vi "FourGaussiansNlin.vi"() -> ()   [LabVIEW 2015]
uses:
  <vilib>/gmath/NumericalOptimization/Nonlinear Curve Fit LM.vi
  <vilib>/gmath/NI_Gmath.lvlib
panel:
  out "array":dbl[][](array[numeric])
  out "error out":errorcluster
  in  "Parameter Guess":dbl[][](array[numeric])=[[1.0, 3224.0, 82.8], [1.0, 3280.0, 64.0], [1.0, 3480.0, 40.0], [1.0, 3518.0, 40.0]] caption="Amplitude     Position        Width" format="%.2f"
  out "Results":string[][](table)
  out "Fit":cluster{dbl, dbl, dbl[][]}(graph)
  # "Initial Guesses (add or remove rows as needed)"
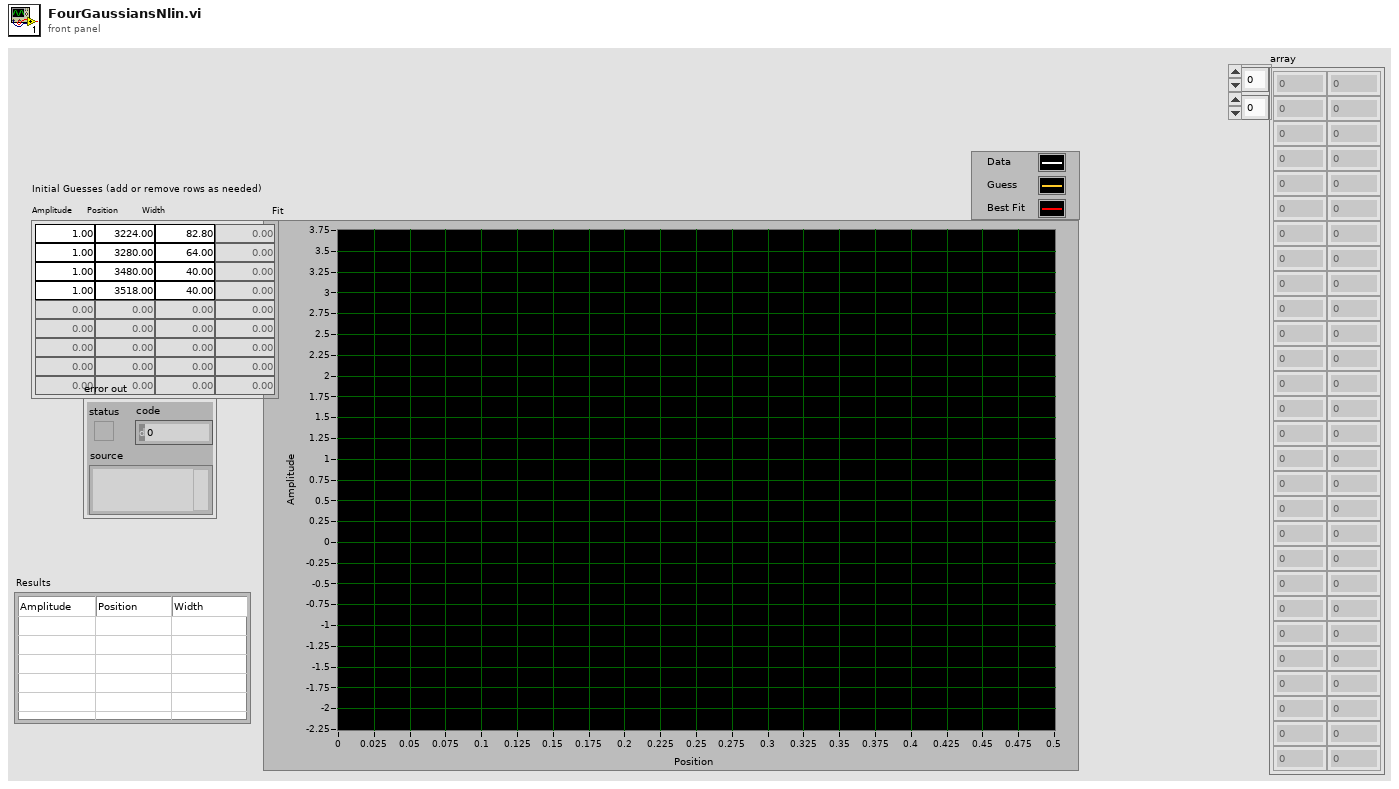
[diagram p1: front panel]
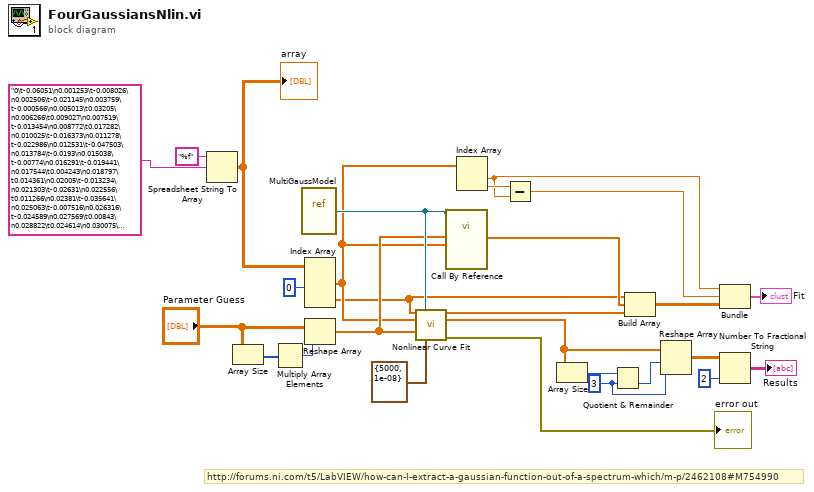
[diagram p0: block diagram]
diagram:
  w4 = 3 ("y")
  # "http://forums.ni.com/t5/LabVIEW/how-can-I-extract-a-gaussian-function-out-of-a-spectrum-which/m-p/2462108#M754990"
  n1 = Spreadsheet String To Array(format string="%f", spreadsheet string="0\t-0.06051\n0.001253\t-0.008026\n0.002506\t-0.021145\n0.003759\t-0.000566\n0.005013\t0.03205\n0.006266\t0.009027\n0.007519\t-0.013454\n0.008772\t0.017282\n0.010025\t-0.016373\n0.011278\t-0.022986\n0.012531\t-0.047503\n0.013784\t-0.0193\n0.015038\t-0.00774\n0.016291\t-0.019441\n0.017544\t0.004243\n0.018797\t0.014361\n0.02005\t-0.013234\n0.021303\t-0.02631\n0.022556\t0.011266\n0.02381\t-0.035641\n0.025063\t-0.007516\n0.026316\t-0.024589\n0.027569\t0.00843\n0.028822\t0.024614\n0.030075\t-0.045957\n0.031328\t-0.057716\n0.032581\t-0.043953\n0.033835\t-0.031529\n0.035088\t-0.081927\n0.036341\t-0.091408\n0.037594\t-0.098195\n0.038847\t-0.089564\n0.0401\t-0.038276\n0.041353\t-0.08202\n0.042607\t-0.091543\n0.04386\t-0.046757\n0.045113\t-0.09163\n0.046366\t-0.088749\n0.047619\t-0.064658\n0.048872\t-0.072261\n0.050125\t-0.12707\n0.051378\t-0.104708\n0.052632\t-0.103939\n0.053885\t-0.093157\n0.055138\t-0.132049\n0.056391\t-0.114817\n0.057644\t-0.121724\n0.058897\t-0.104782\n0.06015\t-0.142024\n0.061404\t-0.131957\n0.062657\t-0.176914\n0.06391\t-0.161334\n0.065163\t-0.14284\n0.066416\t-0.156644\n0.067669\t-0.201751\n0.068922\t-0.166965\n0.070175\t-0.188029\n0.071429\t-0.205835\n0.072682\t-0.272606\n0.073935\t-0.278951\n0.075188\t-0.27726\n0.076441\t-0.258719\n0.077694\t-0.230262\n0.078947\t-0.27264\n0.080201\t-0.295268\n0.081454\t-0.247801\n0.082707\t-0.284363\n0.08396\t-0.305459\n0.085213\t-0.322454\n0.086466\t-0.321781\n0.087719\t-0.361286\n0.088972\t-0.333156\n0.090226\t-0.348285\n0.091479\t-0.358595\n0.092732\t-0.39051\n0.093985\t-0.382925\n0.095238\t-0.491624\n0.096491\t-0.463605\n0.097744\t-0.462484\n0.098997\t-0.470019\n0.100251\t-0.469667\n0.101504\t-0.517955\n0.102757\t-0.59736\n0.10401\t-0.584936\n0.105263\t-0.577842\n0.106516\t-0.609382\n0.107769\t-0.595847\n0.109023\t-0.654391\n0.110276\t-0.651756\n0.111529\t-0.684239\n0.112782\t-0.675556\n0.114035\t-0.72925\n0.115288\t-0.712574\n0.116541\t-0.764648\n0.117794\t-0.74467\n0.119048\t-0.77396\n0.120301\t-0.829208\n0.121554\t-0.85807\n0.122807\t-0.902266\n0.12406\t-0.932697\n0.125313\t-0.898871\n0.126566\t-1.022656\n0.12782\t-0.929653\n0.129073\t-0.990668\n0.130326\t-1.016715\n0.131579\t-1.062086\n0.132832\t-1.088136\n0.134085\t-1.090147\n0.135338\t-1.178622\n0.136591\t-1.189203\n0.137845\t-1.158555\n0.139098\t-1.221042\n0.140351\t-1.225178\n0.141604\t-1.249981\n0.142857\t-1.296073\n0.14411\t-1.285886\n0.145363\t-1.310712\n0.146617\t-1.362254\n0.14787\t-1.366437\n0.149123\t-1.374629\n0.150376\t-1.408814\n0.151629\t-1.418909\n0.152882\t-1.461478\n0.154135\t-1.498747\n0.155388\t-1.530223\n0.156642\t-1.482521\n0.157895\t-1.561413\n0.159148\t-1.559136\n0.160401\t-1.651416\n0.161654\t-1.656585\n0.162907\t-1.606711\n0.16416\t-1.648703\n0.165414\t-1.657518\n0.166667\t-1.70666\n0.16792\t-1.780643\n0.169173\t-1.690411\n0.170426\t-1.798746\n0.171679\t-1.788852\n0.172932\t-1.84627\n0.174185\t-1.843477\n0.175439\t-1.833331\n0.176692\t-1.885198\n0.177945\t-1.887675\n0.179198\t-1.924923\n0.180451\t-1.874285\n0.181704\t-1.901879\n0.182957\t-1.907824\n0.184211\t-1.94076\n0.185464\t-1.952966\n0.186717\t-1.978324\n0.18797\t-1.97581\n0.189223\t-1.949066\n0.190476\t-2.007462\n0.191729\t-2.003745\n0.192982\t-2.002412\n0.194236\t-1.954237\n0.195489\t-1.968438\n0.196742\t-1.992692\n0.197995\t-1.998839\n0.199248\t-1.989507\n0.200501\t-1.948727\n0.201754\t-1.963294\n0.203008\t-1.96246\n0.204261\t-1.987921\n0.205514\t-1.928685\n0.206767\t-1.96992\n0.20802\t-1.970377\n0.209273\t-1.925754\n0.210526\t-1.920443\n0.211779\t-1.931008\n0.213033\t-1.875866\n0.214286\t-1.873133\n0.215539\t-1.870405\n0.216792\t-1.831801\n0.218045\t-1.81055\n0.219298\t-1.786656\n0.220551\t-1.794961\n0.221805\t-1.735744\n0.223058\t-1.733951\n0.224311\t-1.656869\n0.225564\t-1.640512\n0.226817\t-1.569638\n0.22807\t-1.556173\n0.229323\t-1.553107\n0.230576\t-1.493865\n0.23183\t-1.458722\n0.233083\t-1.369252\n0.234336\t-1.357504\n0.235589\t-1.262325\n0.236842\t-1.158763\n0.238095\t-1.126843\n0.239348\t-1.098735\n0.240602\t-1.046933\n0.241855\t-1.012666\n0.243108\t-0.862027\n0.244361\t-0.823745\n0.245614\t-0.699202\n0.246867\t-0.688505\n0.24812\t-0.557859\n0.249373\t-0.466336\n0.250627\t-0.3712\n0.25188\t-0.224461\n0.253133\t-0.156493\n0.254386\t-0.106922\n0.255639\t0.011941\n0.256892\t0.161836\n0.258145\t0.282987\n0.259398\t0.405242\n0.260652\t0.480222\n0.261905\t0.634988\n0.263158\t0.742301\n0.264411\t0.893291\n0.265664\t0.992733\n0.266917\t1.120658\n0.26817\t1.214356\n0.269424\t1.378018\n0.270677\t1.500175\n0.27193\t1.580014\n0.273183\t1.754763\n0.274436\t1.88269\n0.275689\t2.018036\n0.276942\t2.097961\n0.278195\t2.261037\n0.279449\t2.361972\n0.280702\t2.436227\n0.281955\t2.537223\n0.283208\t2.691502\n0.284461\t2.723556\n0.285714\t2.854652\n0.286967\t2.934386\n0.288221\t3.006192\n0.289474\t3.114692\n0.290727\t3.210022\n0.29198\t3.229061\n0.293233\t3.297714\n0.294486\t3.367713\n0.295739\t3.39544\n0.296992\t3.399266\n0.298246\t3.421329\n0.299499\t3.492921\n0.300752\t3.491914\n0.302005\t3.538588\n0.303258\t3.486825\n0.304511\t3.478616\n0.305764\t3.538698\n0.307018\t3.474211\n0.308271\t3.471053\n0.309524\t3.437309\n0.310777\t3.391684\n0.31203\t3.2891\n0.313283\t3.270193\n0.314536\t3.254173\n0.315789\t3.161727\n0.317043\t3.110526\n0.318296\t3.04256\n0.319549\t2.954129\n0.320802\t2.854293\n0.322055\t2.817455\n0.323308\t2.756881\n0.324561\t2.657617\n0.325815\t2.530676\n0.327068\t2.472321\n0.328321\t2.369514\n0.329574\t2.276228\n0.330827\t2.191425\n0.33208\t2.105197\n0.333333\t1.999776\n0.334586\t1.933587\n0.33584\t1.790085\n0.337093\t1.709929\n0.338346\t1.606816\n0.339599\t1.569115\n0.340852\t1.467204\n0.342105\t1.374485\n0.343358\t1.271246\n0.344612\t1.208708\n0.345865\t1.146691\n0.347118\t1.067424\n0.348371\t1.026071\n0.349624\t0.947353\n0.350877\t0.848002\n0.35213\t0.817193\n0.353383\t0.737234\n0.354637\t0.660038\n0.35589\t0.635437\n0.357143\t0.621938\n0.358396\t0.510392\n0.359649\t0.468965\n0.360902\t0.430646\n0.362155\t0.434983\n0.363409\t0.374562\n0.364662\t0.349808\n0.365915\t0.315216\n0.367168\t0.26208\n0.368421\t0.23222\n0.369674\t0.261424\n0.370927\t0.198689\n0.37218\t0.163642\n0.373434\t0.180502\n0.374687\t0.141132\n0.37594\t0.149584\n0.377193\t0.091697\n0.378446\t0.133451\n0.379699\t0.048741\n0.380952\t0.065287\n0.382206\t0.080531\n0.383459\t0.029787\n0.384712\t0.047321\n0.385965\t0.087086\n0.387218\t0.013222\n0.388471\t0.040555\n0.389724\t0.035707\n0.390977\t0.021196\n0.392231\t0.016688\n0.393484\t0.04938\n0.394737\t0.043507\n0.39599\t-0.051322\n0.397243\t0.021564\n0.398496\t-0.012005\n0.399749\t0.015103\n0.401003\t0.046354\n0.402256\t-0.04566\n0.403509\t0.018695\n0.404762\t-0.021761\n0.406015\t0.007368\n0.407268\t0.018921\n0.408521\t0.003829\n0.409774\t-0.004485\n0.411028\t0.019233\n0.412281\t0.023709\n0.413534\t0.027282\n0.414787\t-0.019432\n0.41604\t0.049524\n0.417293\t0.024324\n0.418546\t-0.001887\n0.419799\t0.006426\n0.421053\t-0.01426\n0.422306\t0.024085\n0.423559\t0.039121\n0.424812\t-0.010473\n0.426065\t-0.009608\n0.427318\t0.005581\n0.428571\t-0.018264\n0.429825\t0.023284\n0.431078\t0.02597\n0.432331\t-0.022661\n0.433584\t0.016826\n0.434837\t-0.029228\n0.43609\t-0.006769\n0.437343\t-0.029571\n0.438596\t0.028512\n0.43985\t-0.014078\n0.441103\t0.046834\n0.442356\t0.023905\n0.443609\t0.016553\n0.444862\t-0.029599\n0.446115\t0.000861\n0.447368\t-0.019257\n0.448622\t0.010707\n0.449875\t-0.022876\n0.451128\t0.022984\n0.452381\t0.051314\n0.453634\t0.012523\n0.454887\t-0.002974\n0.45614\t0.020154\n0.457393\t0.006899\n0.458647\t-0.032641\n0.4599\t-0.005378\n0.461153\t-0.044238\n0.462406\t-0.051467\n0.463659\t-0.008786\n0.464912\t0.009103\n0.466165\t-0.041656\n0.467419\t0.026368\n0.468672\t0.000754\n0.469925\t-0.042104\n0.471178\t-0.022092\n0.472431\t-0.027057\n0.473684\t0.003766\n0.474937\t0.043316\n0.47619\t-0.054678\n0.477444\t0.001355\n0.478697\t-0.02857\n0.47995\t0.020187\n0.481203\t-0.019112\n0.482456\t0.014614\n0.483709\t-0.005761\n0.484962\t-0.048509\n0.486216\t0.022678\n0.487469\t-0.003371\n0.488722\t0.000941\n0.489975\t0.004019\n0.491228\t0.000624\n0.492481\t-0.026588\n0.493734\t-0.042389\n0.494987\t-0.016744\n0.496241\t0.04837\n0.497494\t-0.004465\n0.498747\t0.007572\n0.5\t-0.017557") -> (array=w18:dbl[][])  [unwired: 2 in]
  "array" <- w18
  n2 = Array Size(array="Parameter Guess") -> (size(s)=w25:i32[])
  n3 = Multiply Array Elements(1:w25) -> (0:w24:i32)
  n4 = vi-ref "MultiGaussModel.vi"() -> (w22:refnum<vi>)
  n5 = Index Array(array=w18, index (col) #1=0 ("disabled index (col)")) -> (element #1=w16:dbl[], element #2=w11:dbl[])  [unwired: 3 in]
  n6 = Reshape Array("Parameter Guess", w24) -> (w21:dbl[])
  n7 = call-poly <vilib>:"Nonlinear Curve Fit.vi"("Y"=w11, "f(x,a)"=w22, "X"=w16, "initial parameters"=w21, "termination"=cluster{"max iteration":i32, "tolerance":dbl} {"max iteration"=5000, "tolerance"=1e-08}) -> ("best nonlinear fit"=w9:dbl[], "best fit parameters"=w2:dbl[], "error out"=→"error out":errorcluster)  [unwired: 5 in, 3 out]
  n8 = call-by-ref "?"(reference=w22, "X"=w16, "a"=w21) -> ("f(X,a)"=w12:dbl[])  [unwired: 3 in, 4 out]
  n9 = Index Array(array=w16) -> (element #1=w14:dbl, element #2=w15:dbl)  [unwired: 2 in]
  n10 = Subtract(x=w15, y=w14) -> (x-y=w13:dbl)
  n11 = Array Size(array=w2) -> (size(s)=w3:i32)
  n12 = Quotient & Remainder(x=w3, y=w4) -> (floor(x/y)=w5:i32)  [unwired: 1 out]
  n13 = Build Array(w11, w12, w9) -> (w27:dbl[][])
  n14 = Reshape Array(w2, w5, w4) -> (w1:dbl[][])
  n15 = Bundle(w14, w13, w27) -> (→"Fit":cluster{dbl, dbl, dbl[][]})  [unwired: 1 in]
  n16 = Number To Fractional String(number=w1, precision (6)=i16 2) -> (F-format string=→"Results":string[][])  [unwired: 2 in]
